vi "DemoWriteAnalog.vi"   [LabVIEW 2009]
uses:
  <vilib>/NXT/Block Support/NXT_InputPort.ctl
  <vilib>/NXT/Dual Mode Library/Waits/Wait_Num(msec).vi
panel:
  # "Demo Analog Write"
types:
  T1 = typedef "NXT_InputPort.ctl" = u8
  T2 = typedef "LVHSConnector.ctl" = cluster{"error":errorcluster, "address":string, "NXT #":i32, "Show Error":bool, "Connection":u16}
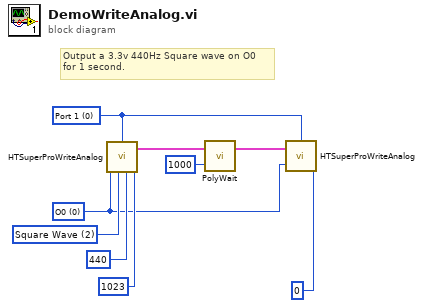
[diagram p0: block diagram]
diagram:
  w2 = u8 0 items=["O0", "O1"] ("Analog Output")
  w7 = u8 2 items=["DC", "Sine Wave", "Square Wave", "Pos Sawtooth Wave", "Neg Sawtooth Wave", "Triangle Wave", "PWM Voltage"] ("Analog Mode")
  w3 = T1 0 items=["Port 1", "Port 2", "Port 3", "Port 4"] ("Port")
  # "Output a 3.3v 440Hz Square wave on O0\nfor 1 second."
  n1 = call "HTSuperProWriteAnalog.vi"("Port"=w3, "Voltage"=i16 1023, "Frequency"=i16 440, "Analog Mode"=w7, "Analog Output"=w2) -> ("NXT"=w8:T2)  [unwired: 1 in]
  n2 = call-poly <vilib>:"PolyWait.vi"("Time (100 msec)"=u32 1000, "NXT"=w8) -> ("NXT"=w4:T2)  [unwired: 2 in]
  n3 = call "HTSuperProWriteAnalog.vi"("Port"=w3, "NXT"=w4, "Voltage"=i16 0, "Analog Output"=w2) -> ()  [unwired: 2 in, 1 out]
